vi "correctormicras.vi"(6 "paso":dbl, 8 "x fin.":dbl, 9 "y fin.":dbl, 10 "y inic.":dbl, 11 "x inic.":dbl) -> (0 "y fin sal.":dbl, 1 "x finsalida":dbl, 2 "y inic.sal":dbl, 3 "x inic.sal":dbl, 5 "paso sal":dbl)   [LabVIEW 2016]
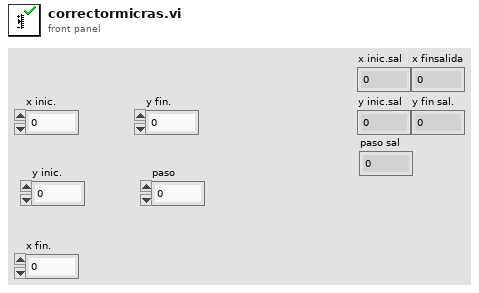
[diagram p1: front panel]
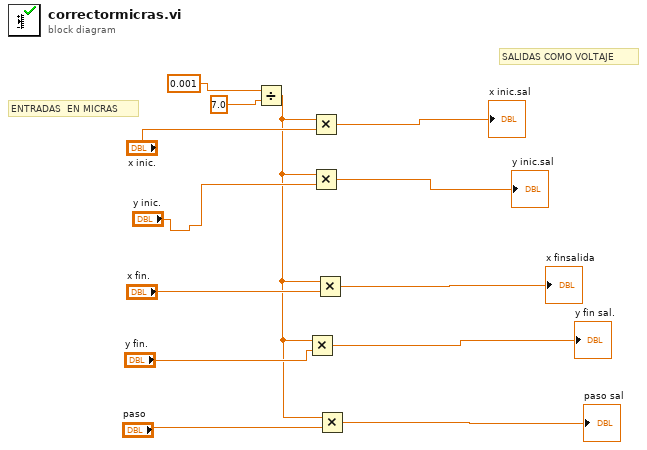
[diagram p0: block diagram]
diagram:
  # "ENTRADAS  EN MICRAS"
  # "SALIDAS COMO VOLTAJE"
  n1 = Divide(x=0.001 ("y"), y=7.0) -> (x/y=w6:dbl)
  n2 = Multiply(x=w6, y="y fin.") -> (x*y=→"y fin sal.":dbl)
  n3 = Multiply(x=w6, y="x inic.") -> (x*y=→"x inic.sal":dbl)
  n4 = Multiply(x=w6, y="y inic.") -> (x*y=→"y inic.sal":dbl)
  n5 = Multiply(x=w6, y="x fin.") -> (x*y=→"x finsalida":dbl)
  n6 = Multiply(x=w6, y="paso") -> (x*y=→"paso sal":dbl)
